vi "Build Packed Libraries.vi"(8 "Changes":string, 9 "Build Options":T2, 10 "Version Increment":T3, 11 "Calling VI References":T1) -> (3 "Build Error":bool)   [LabVIEW 2021, in "TemplateCoreUtilities.lvlib"]
uses:
  TemplateCoreUtilities.lvlib
  <vilib>/CIF Foundation/CIF LabVIEW Scripting/LV Scripting/Typedef/Version Increment.ctl
  Typedef/Build Options.ctl
  Typedef/Calling VI References.ctl
  <vilib>/CIF Foundation/CIF LabVIEW Scripting/LV Scripting/Typedef/Version.ctl
  <vilib>/CIF Foundation/CIF Core/CIFUtilities/Scripting/Build Libraries/LabVIEW Build Script/LabVIEW Build Script.lvclass/LabVIEW Build Script.ctl
  <vilib>/CIF Foundation/CIF LabVIEW Scripting/LV Scripting/SubVIs/Add Scripting Error.vi
  <vilib>/CIF Foundation/CIF Utilities/Errors/Append Error Location.vi
  <vilib>/AppBuilder/AB_API_Simple/Build (path).vi
  <vilib>/CIF Foundation/CIF Core/CIFUtilities/Scripting/Build Libraries/LabVIEW Build Script/LabVIEW Build Script.lvclass
  <vilib>/CIF Foundation/CIF LabVIEW Scripting/LV Scripting/LV Scripting Utilities.lvlib
  <vilib>/AppBuilder/AB_API_Simple/NI_App_Builder_API.lvlib
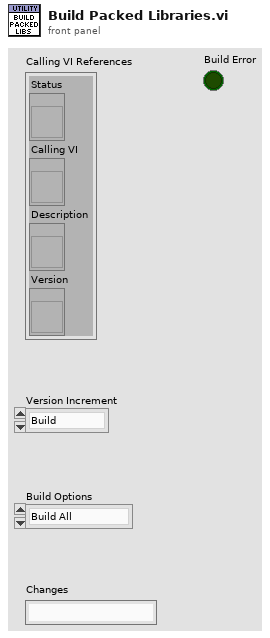
[diagram p1: front panel]
types:
  T1 = typedef "TemplateCoreUtilities.lvlib/Calling VI References.ctl" = cluster{"Status":refnum<vi>, "Calling VI":refnum<vi>, "Description":refnum<vi>, "Version":refnum<vi>}
  T2 = typedef "TemplateCoreUtilities.lvlib/Build Options.ctl" = enum16{"Build All", "Build RT Only", "Build Win Only", "Build UI Only"}
  T3 = typedef "LV Scripting Utilities.lvlib/Version Increment.ctl" = enum16{"Build", "Fix", "Minor", "Major"}
  T4 = typedef "Version.ctl" = cluster{"Major":u16, "Minor":u16, "Fix":u16, "Build":u16}
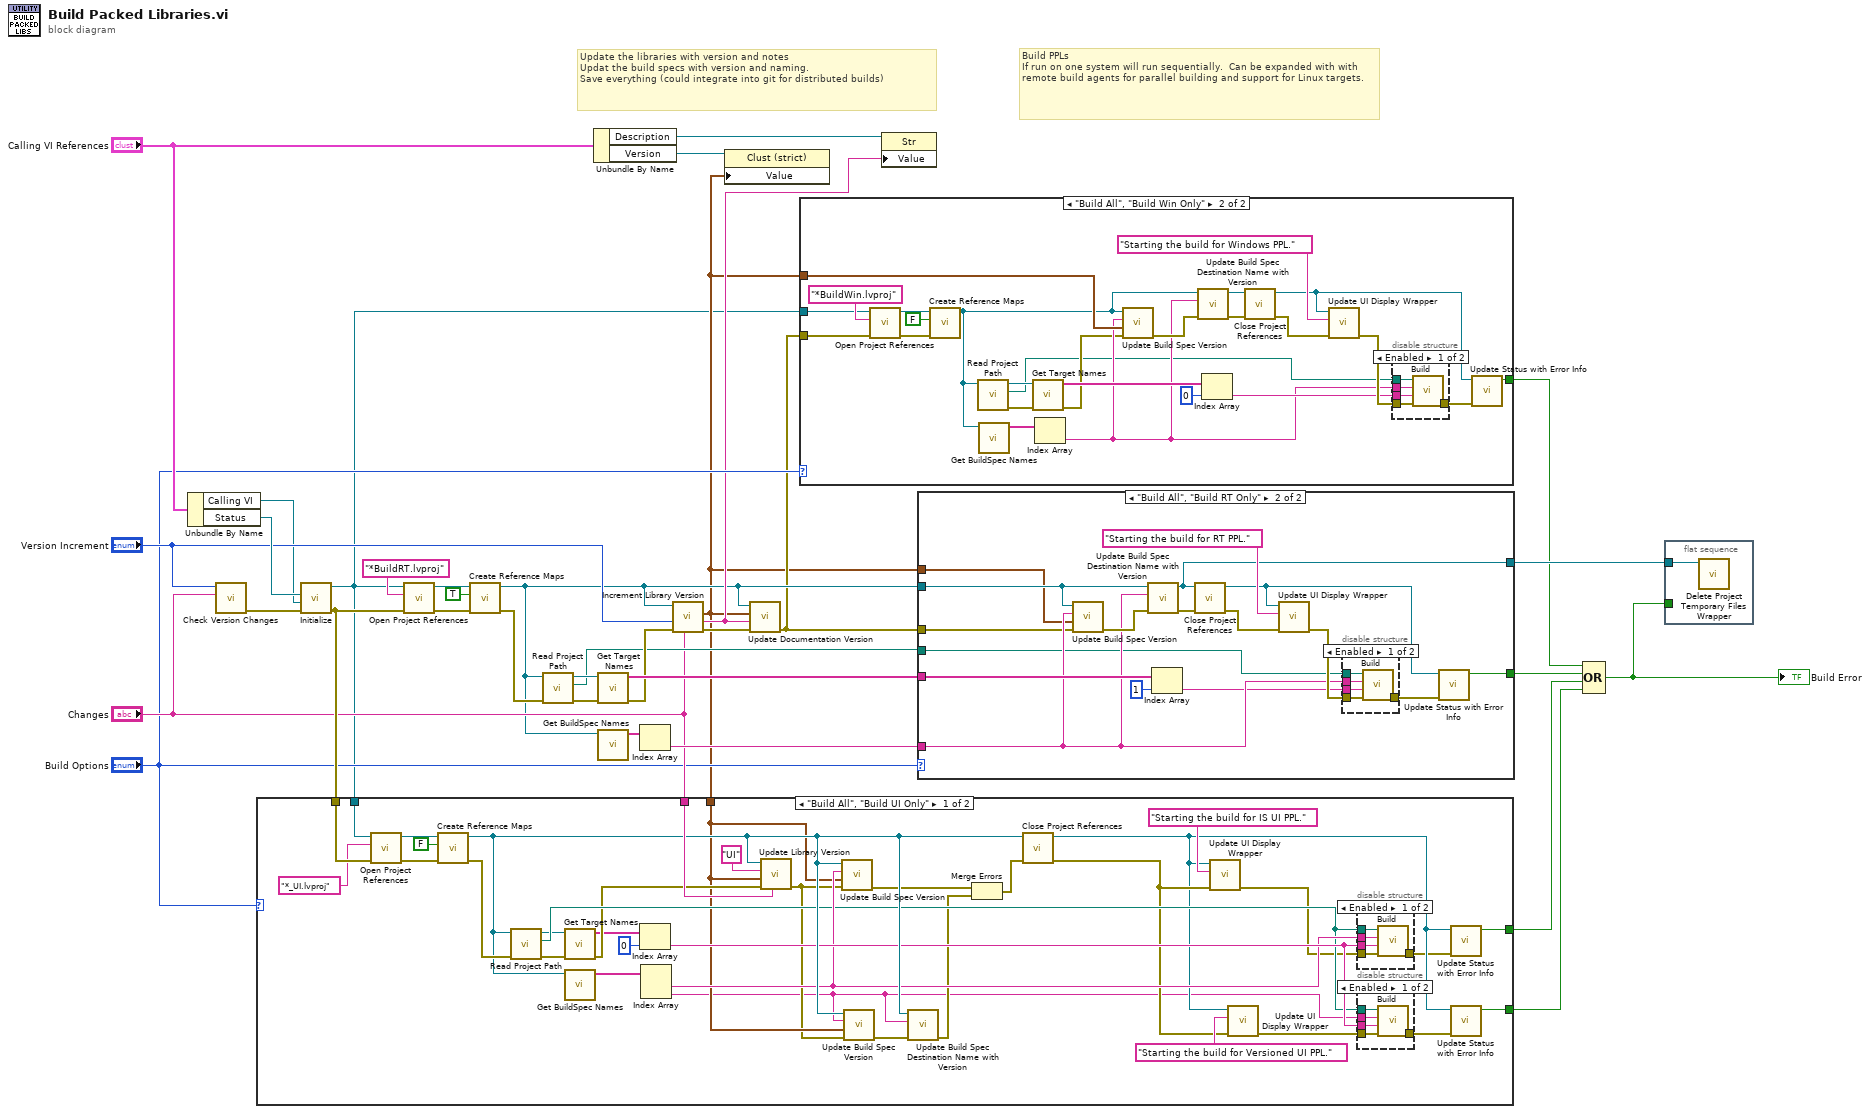
[diagram p0: block diagram]
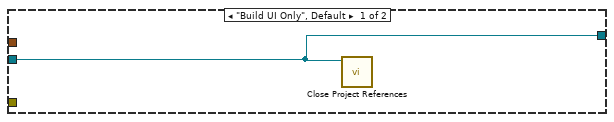
[diagram p4: hidden frame]
diagram:
  # "Build PPLs\nIf run on one system will run sequentially.  Can be expanded with with remote build agents for parallel building and support for Linux targets."
  # "Update the libraries with version and notes\nUpdat the build specs with version and naming.\nSave everything (could integrate into git for distributed builds)"
  n1 = Unbundle By Name("Calling VI References") -> ("Calling VI"=w12:refnum<vi>, "Status"=w17:refnum<vi>)
  n2 = call <vilib>:"Check Version Changes.vi"("Changes"="Changes", "Version Increment"="Version Increment") -> ("error out"=w32:errorcluster)  [unwired: 9 in]
  n3 = call <vilib>:"Initialize.vi"("error in (no error)"=w32, "Calling VI"=w12, "UI Display"=w17) -> ("error out"=w34:errorcluster, "LabVIEW Build Script out"=w1:refnum<class "LabVIEW Build Script.lvclass">)  [unwired: 7 in]
  n4 = call <vilib>:"Open Project References.vi"("error in (no error)"=w34, "Search Pattern"="*BuildRT.lvproj" ("pattern"), "LabVIEW Build Script in"=w1) -> ("error out"=w30:errorcluster, "LabVIEW Build Script out"=w29:refnum<class "LabVIEW Build Script.lvclass">)  [unwired: 7 in]
  n5 = call <vilib>:"Create Reference Maps.vi"("error in (no error)"=w30, "RT Target"=TRUE, "LabVIEW Build Script in"=w29) -> ("error out"=w33:errorcluster, "LabVIEW Build Script out"=w4:refnum<class "LabVIEW Build Script.lvclass">)  [unwired: 7 in]
  n6 = call <vilib>:"Read Project Path.vi"("error in (no error)"=w33, "LabVIEW Build Script in"=w4) -> ("error out"=w26:errorcluster, "Project Path"=w21:path, "LabVIEW Build Script out"=w27:refnum<class "LabVIEW Build Script.lvclass">)  [unwired: 7 in]
  n7 = Unbundle By Name("Calling VI References") -> ("Description"=w14:refnum<vi>, "Version"=w15:refnum<vi>)
  n8 = call <vilib>:"Get Target Names.vi"("error in (no error)"=w26, "LabVIEW Build Script in"=w27) -> ("error out"=w23:errorcluster, "Project Targets"=w25:string[])  [unwired: 8 in]
  n9 = call <vilib>:"Get BuildSpec Names.vi"("LabVIEW Build Script in"=w4) -> ("BuildSpecs"=w24:string[])  [unwired: 10 in]
  n10 = Index Array(array=w24) -> (element=w22:string)  [unwired: 1 in]
  n11 = call <vilib>:"Increment Library Version.vi"("Changes"="Changes", "error in (no error)"=w23, "Version Increment"="Version Increment", "LabVIEW Build Script in"=w4) -> ("error out"=w6:errorcluster, "Description"=w5:string, "Version"=w2:T4)  [unwired: 5 in]
  n12 = case shown="\"Build All\", \"Build UI Only\"" "Build Options" {
    tunnel: w34 -> [w70 _]
    tunnel: w1 -> [w35 _]
    tunnel: "Changes" -> [w69 _]
    tunnel: [w62 _] -> w19
    tunnel: [w61 _] -> w18
    tunnel: w2 -> [w44 _]
    frame "Build All", "Build UI Only" {
      n13 = call <vilib>:"Open Project References.vi"("error in (no error)"=w70, "Search Pattern"="*_UI.lvproj" ("pattern"), "LabVIEW Build Script in"=w35) -> ("error out"=w68:errorcluster, "LabVIEW Build Script out"=w67:refnum<class "LabVIEW Build Script.lvclass">)  [unwired: 7 in]
      n14 = call <vilib>:"Create Reference Maps.vi"("error in (no error)"=w68, "RT Target"=FALSE, "LabVIEW Build Script in"=w67) -> ("error out"=w65:errorcluster, "LabVIEW Build Script out"=w63:refnum<class "LabVIEW Build Script.lvclass">)  [unwired: 7 in]
      n15 = call <vilib>:"Read Project Path.vi"("error in (no error)"=w65, "LabVIEW Build Script in"=w63) -> ("error out"=w48:errorcluster, "Project Path"=w58:path, "LabVIEW Build Script out"=w47:refnum<class "LabVIEW Build Script.lvclass">)  [unwired: 7 in]
      n16 = call <vilib>:"Get Target Names.vi"("error in (no error)"=w48, "LabVIEW Build Script in"=w47) -> ("error out"=w52:errorcluster, "Project Targets"=w50:string[])  [unwired: 8 in]
      n17 = call <vilib>:"Get BuildSpec Names.vi"("LabVIEW Build Script in"=w63) -> ("BuildSpecs"=w51:string[])  [unwired: 10 in]
      n18 = Index Array(array=w50, index=0) -> (element=w60:string)
      n19 = Index Array(array=w51) -> (element #1=w59:string, element #2=w38:string)  [unwired: 2 in]
      n20 = call <vilib>:"Update Library Version.vi"("Changes"=w69, "error in (no error)"=w52, "Version"=w44, "Search Pattern"="UI", "LabVIEW Build Script in"=w63) -> ("error out"=w40:errorcluster)  [unwired: 5 in, 1 out]
      n21 = call <vilib>:"Update Build Spec Version.vi"("error in (no error)"=w40, "Version"=w44, "Search Pattern"=w59, "LabVIEW Build Script in"=w63) -> ("error out"=w43:errorcluster)  [unwired: 7 in]
      n22 = call <vilib>:"Update Build Spec Version.vi"("error in (no error)"=w40, "Version"=w44, "Search Pattern"=w38, "LabVIEW Build Script in"=w63) -> ("error out"=w54:errorcluster)  [unwired: 7 in]
      n23 = call <vilib>:"Update Build Spec Destination Name with Version.vi"("error in (no error)"=w54, "Search Pattern"=w38, "LabVIEW Build Script in"=w63) -> ("error out"=w42:errorcluster)  [unwired: 7 in, 1 out]
      n24 = Merge Errors(w43, w42) -> (w41:errorcluster)
      n25 = call <vilib>:"Close Project References.vi"("error in (no error)"=w41, "LabVIEW Build Script in"=w63) -> ("error out"=w56:errorcluster, "LabVIEW Build Script out"=w45:refnum<class "LabVIEW Build Script.lvclass">)  [unwired: 8 in]
      n26 = call <vilib>:"Update UI Display Wrapper.vi"("error in (no error)"=w56, "Update for Display"="Starting the build for IS UI PPL.", "LabVIEW Build Script in"=w45) -> ("error out"=w53:errorcluster)  [unwired: 8 in]
      n27 = call <vilib>:"Update UI Display Wrapper.vi"("error in (no error)"=w56, "Update for Display"="Starting the build for Versioned UI PPL.", "LabVIEW Build Script in"=w45) -> ("error out"=w37:errorcluster)  [unwired: 8 in]
      n28 = disable-structure shown="Enabled" {
        disable-tunnel: w58 -> [w81 _]
        disable-tunnel: w60 -> [w80 _]
        disable-tunnel: w59 -> [w79 _]
        disable-tunnel: w53 -> [w78 w82]
        disable-tunnel: [w77 w82] -> w39
        frame Enabled {
          n29 = call-poly <vilib>:"Build.vi"("error in (no error)"=w78, "Name of target (My Computer)"=w80, "Name of build specification (if empty: build all)"=w79, "Path to project"=w81) -> ("error out"=w77:errorcluster)  [unwired: 6 in, 1 out]
        }
        frame Disabled {
        }
      }
      n30 = disable-structure shown="Enabled" {
        disable-tunnel: w58 -> [w75 _]
        disable-tunnel: w60 -> [w74 _]
        disable-tunnel: w38 -> [w73 _]
        disable-tunnel: w37 -> [w72 w76]
        disable-tunnel: [w71 w76] -> w46
        frame Enabled {
          n31 = call-poly <vilib>:"Build.vi"("error in (no error)"=w72, "Name of target (My Computer)"=w74, "Name of build specification (if empty: build all)"=w73, "Path to project"=w75) -> ("error out"=w71:errorcluster)  [unwired: 6 in, 1 out]
        }
        frame Disabled {
        }
      }
      n32 = call <vilib>:"Update Status with Error Info.vi"("error in (no error)"=w39, "LabVIEW Build Script"=w45) -> ("Error"=w62:bool)  [unwired: 9 in]
      n33 = call <vilib>:"Update Status with Error Info.vi"("error in (no error)"=w46, "LabVIEW Build Script"=w45) -> ("Error"=w61:bool)  [unwired: 9 in]
    }
    frame "Build RT Only", Default {
    }
  }
  n34 = property class="Clust (strict)"(reference=w15, "Value"=w2) -> ()  [unwired: 1 in, 2 out]
  n35 = call <vilib>:"Update Documentation Version.vi"("error in (no error)"=w6, "Description"=w5, "Version"=w2, "LabVIEW Build Script in"=w4) -> ("error out"=w3:errorcluster)  [unwired: 7 in]
  n36 = case shown="\"Build All\", \"Build Win Only\"" "Build Options" {
    tunnel: w3 -> [_ w96]
    tunnel: [_ w100] -> w7
    tunnel: w2 -> [_ w99]
    tunnel: w1 -> [_ w83]
    frame "Build UI Only", Default {
    }
    frame "Build All", "Build Win Only" {
      n37 = call <vilib>:"Open Project References.vi"("error in (no error)"=w96, "Search Pattern"="*BuildWin.lvproj" ("pattern"), "LabVIEW Build Script in"=w83) -> ("error out"=w93:errorcluster, "LabVIEW Build Script out"=w94:refnum<class "LabVIEW Build Script.lvclass">)  [unwired: 7 in]
      n38 = call <vilib>:"Create Reference Maps.vi"("error in (no error)"=w93, "RT Target"=FALSE, "LabVIEW Build Script in"=w94) -> ("LabVIEW Build Script out"=w84:refnum<class "LabVIEW Build Script.lvclass">)  [unwired: 7 in, 1 out]
      n39 = call <vilib>:"Read Project Path.vi"("LabVIEW Build Script in"=w84) -> ("error out"=w91:errorcluster, "Project Path"=w86:path, "LabVIEW Build Script out"=w90:refnum<class "LabVIEW Build Script.lvclass">)  [unwired: 8 in]
      n40 = call <vilib>:"Get BuildSpec Names.vi"("LabVIEW Build Script in"=w84) -> ("BuildSpecs"=w92:string[])  [unwired: 10 in]
      n41 = call <vilib>:"Get Target Names.vi"("error in (no error)"=w91, "LabVIEW Build Script in"=w90) -> ("error out"=w87:errorcluster, "Project Targets"=w89:string[])  [unwired: 8 in]
      n42 = Index Array(array=w92) -> (element=w88:string)  [unwired: 1 in]
      n43 = call <vilib>:"Update Build Spec Version.vi"("error in (no error)"=w87, "Version"=w99, "Search Pattern"=w88, "LabVIEW Build Script in"=w84) -> ("error out"=w104:errorcluster)  [unwired: 7 in]
      n44 = call <vilib>:"Update Build Spec Destination Name with Version.vi"("error in (no error)"=w104, "Search Pattern"=w88, "LabVIEW Build Script in"=w84) -> ("error out"=w105:errorcluster, "LabVIEW Build Script out"=w97:refnum<class "LabVIEW Build Script.lvclass">)  [unwired: 7 in]
      n45 = Index Array(array=w89, index=0) -> (element=w102:string)
      n46 = call <vilib>:"Close Project References.vi"("error in (no error)"=w105, "LabVIEW Build Script in"=w97) -> ("error out"=w107:errorcluster, "LabVIEW Build Script out"=w98:refnum<class "LabVIEW Build Script.lvclass">)  [unwired: 8 in]
      n47 = call <vilib>:"Update UI Display Wrapper.vi"("error in (no error)"=w107, "Update for Display"="Starting the build for Windows PPL.", "LabVIEW Build Script in"=w98) -> ("error out"=w103:errorcluster)  [unwired: 8 in]
      n48 = disable-structure shown="Enabled" {
        disable-tunnel: w86 -> [w113 _]
        disable-tunnel: w102 -> [w112 _]
        disable-tunnel: w88 -> [w111 _]
        disable-tunnel: w103 -> [w110 w114]
        disable-tunnel: [w109 w114] -> w101
        frame Enabled {
          n49 = call-poly <vilib>:"Build.vi"("error in (no error)"=w110, "Name of target (My Computer)"=w112, "Name of build specification (if empty: build all)"=w111, "Path to project"=w113) -> ("error out"=w109:errorcluster)  [unwired: 6 in, 1 out]
        }
        frame Disabled {
        }
      }
      n50 = call <vilib>:"Update Status with Error Info.vi"("error in (no error)"=w101, "LabVIEW Build Script"=w98) -> ("Error"=w100:bool)  [unwired: 9 in]
    }
  }
  n51 = property class="Str"(reference=w14, "Value"=w5) -> ()  [unwired: 1 in, 2 out]
  n52 = case shown="\"Build All\", \"Build RT Only\"" "Build Options" {
    tunnel: w4 -> [w115 w132]
    tunnel: w25 -> [_ w128]
    tunnel: w22 -> [_ w124]
    tunnel: w21 -> [_ w122]
    tunnel: w3 -> [_ w116]
    tunnel: [_ w120] -> w20
    tunnel: w2 -> [_ w119]
    tunnel: [w115 w117] -> w10
    frame "Build UI Only", Default {
      n53 = call <vilib>:"Close Project References.vi"("LabVIEW Build Script in"=w115) -> ()  [unwired: 9 in, 2 out]
    }
    frame "Build All", "Build RT Only" {
      n54 = call <vilib>:"Update Build Spec Version.vi"("error in (no error)"=w116, "Version"=w119, "Search Pattern"=w124, "LabVIEW Build Script in"=w132) -> ("error out"=w126:errorcluster)  [unwired: 7 in]
      n55 = call <vilib>:"Update Build Spec Destination Name with Version.vi"("error in (no error)"=w126, "Search Pattern"=w124, "LabVIEW Build Script in"=w132) -> ("error out"=w127:errorcluster, "LabVIEW Build Script out"=w117:refnum<class "LabVIEW Build Script.lvclass">)  [unwired: 7 in]
      n56 = Index Array(array=w128, index=1) -> (element=w123:string)
      n57 = call <vilib>:"Close Project References.vi"("error in (no error)"=w127, "LabVIEW Build Script in"=w117) -> ("error out"=w130:errorcluster, "LabVIEW Build Script out"=w118:refnum<class "LabVIEW Build Script.lvclass">)  [unwired: 8 in]
      n58 = call <vilib>:"Update UI Display Wrapper.vi"("error in (no error)"=w130, "Update for Display"="Starting the build for RT PPL.", "LabVIEW Build Script in"=w118) -> ("error out"=w125:errorcluster)  [unwired: 8 in]
      n59 = disable-structure shown="Enabled" {
        disable-tunnel: w122 -> [w137 _]
        disable-tunnel: w123 -> [w136 _]
        disable-tunnel: w124 -> [w135 _]
        disable-tunnel: w125 -> [w134 w138]
        disable-tunnel: [w133 w138] -> w121
        frame Enabled {
          n60 = call-poly <vilib>:"Build.vi"("error in (no error)"=w134, "Name of target (My Computer)"=w136, "Name of build specification (if empty: build all)"=w135, "Path to project"=w137) -> ("error out"=w133:errorcluster)  [unwired: 6 in, 1 out]
        }
        frame Disabled {
        }
      }
      n61 = call <vilib>:"Update Status with Error Info.vi"("error in (no error)"=w121, "LabVIEW Build Script"=w118) -> ("Error"=w120:bool)  [unwired: 9 in]
    }
  }
  n62 = Compound Arithmetic op=OR(w7, w20, w19, w18) -> (w9:bool)
  "Build Error" <- w9
  n63 = flat-sequence {
    tunnel: w10 -> [w139]
    tunnel: w9 -> [_]
    frame #0 {
      n64 = call <vilib>:"Delete Project Temporary Files Wrapper.vi"("LabVIEW Build Script in"=w139) -> ()  [unwired: 10 in, 1 out]
    }
  }
